vi "create_feature_studio.vi"(1 "New Feature Studio Name":string, 11 "error in":errorcluster) -> (4 "Device Out":T1, 6 "Comm":T2, 15 "error out":errorcluster)   [LabVIEW 2019]
uses:
  <userlib>/IoT Devices/_subVIs/HTTPComm.ctl
  _SubVI/Cluster.ctl
panel:
  in  "Device In":T1
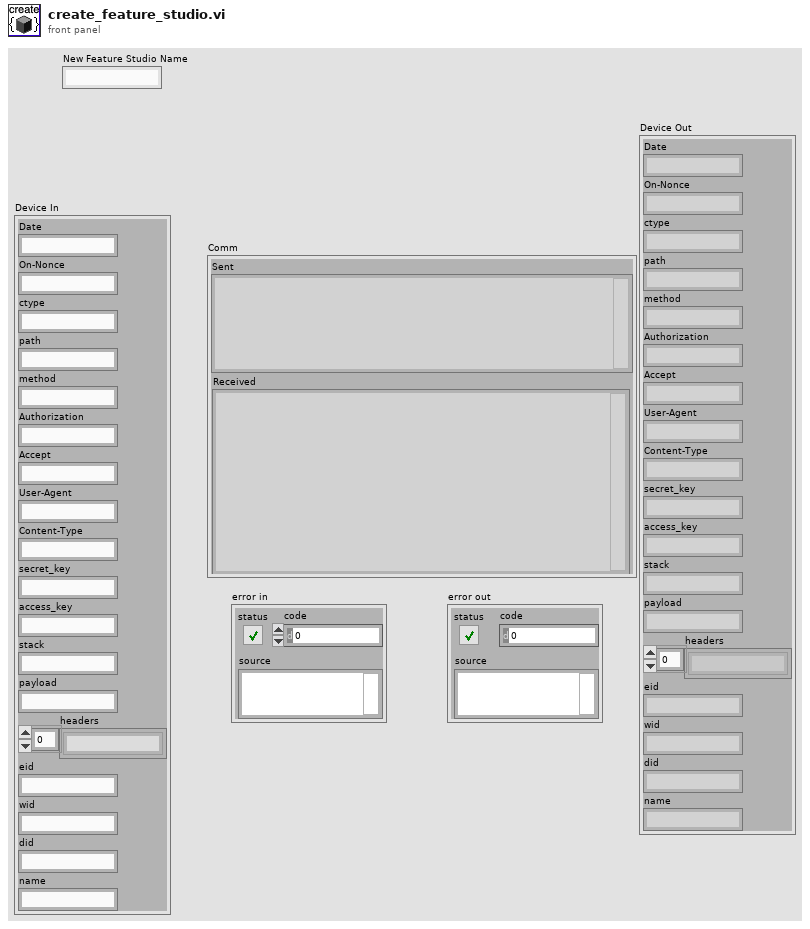
[diagram p1: front panel]
types:
  T1 = typedef "Cluster.ctl" = cluster{"Date":string, "On-Nonce":string, "ctype":string, "path":string, "method":string, "Authorization":string, "Accept":string, "User-Agent":string, "Content-Type":string, "secret_key":string, "access_key":string, "stack":string, "payload":string, "headers":string[], "eid":string, "wid":string, "did":string, "name":string}
  T2 = typedef "HTTPComm.ctl" = cluster{"url":string, "sent headers":string, "sent body":string, "headers":string, "body":string, "Sent":string, "Received":string}
  T3 = cluster{"Date":string, "On-Nonce":string, "ctype":string, "path":string, "method":string, "Authorization":string, "Accept":string, "User-Agent":string, "Content-Type":string, "secret_key":string, "access_key":string, "stack":string, "payload":string, "headers":string[], "eid":string, "wid":string, "did":string, "name":string}
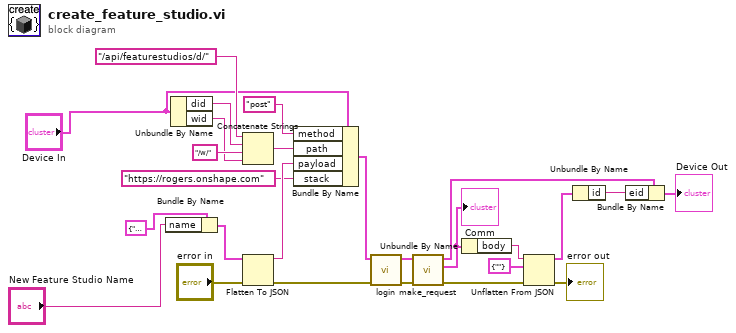
[diagram p0: block diagram]
diagram:
  n1 = Bundle By Name(cluster=cluster{"name":string} {"name"="milan"}, "name"="New Feature Studio Name") -> (w24:cluster{"name":string})
  n2 = Unbundle By Name("Device In") -> ("did"=w15:string, "wid"=w14:string)
  n3 = Concatenate Strings("/api/featurestudios/d/" ("payload"), w15, "/w/" ("string"), w14) -> (w21:string)
  n4 = Flatten To JSON(anything=w24, error in (no error)="error in") -> (JSON string=w20:string, 11:w12:errorcluster)  [unwired: 1 in]
  n5 = Bundle By Name(cluster="Device In", "method"="post" ("Method"), "path"=w21, "payload"=w20, "stack"="https://rogers.onshape.com" ("stacks")) -> (w18:T1)
  n6 = call "login.vi"("error in"=w12, "Device In"=w18) -> ("error out"=w16:errorcluster, "Device Out"=w17:T3)  [unwired: 8 in]
  n7 = call "make_request.vi"("Error in"=w16, "Device In"=w17) -> ("error out"=w2:errorcluster, "Comm"=w8:T2, "Device Out"=w7:T3)  [unwired: 7 in]
  "Comm" <- w8
  n8 = Unbundle By Name(w8) -> ("body"=w9:string)
  n9 = Unflatten From JSON(JSON string=w9, type and defaults=cluster{"id":string} {"id"=""}, error in (no error)=w2) -> (value=w11:cluster{"id":string}, error out=→"error out":errorcluster)  [unwired: 4 in]
  n10 = Unbundle By Name(w11) -> ("id"=w4:string)
  n11 = Bundle By Name(cluster=w7, "eid"=w4) -> (→"Device Out":T3)
